vi "Get Color Ramp.vi"(9 "Number of Colors":i32, 11 "Color Ramp Array":u32[](array[colorbox])) -> (3 "RGB Array":u32[](array[colorbox]))   [LabVIEW 2020, in "3D Plot.lvclass"]
uses:
  <vilib>/Math Plots/3D Math Plots/3D Plot/3D Plot/3D Plot.lvclass
  <vilib>/Utility/colorconv.llb/Color to RGB.vi
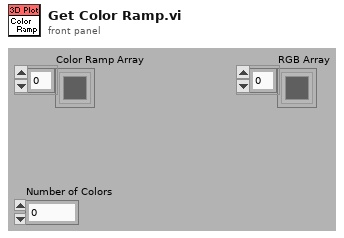
[diagram p1: front panel]
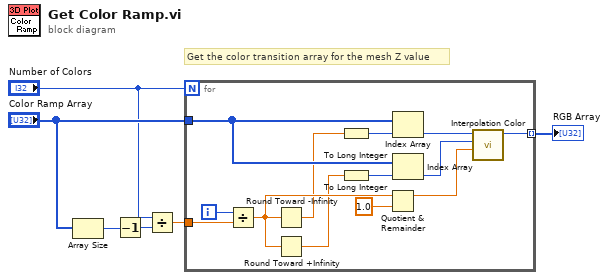
[diagram p0: block diagram]
diagram:
  # "Get the color transition array for the mesh Z value"
  n1 = Array Size(array="Color Ramp Array") -> (size(s)=w5:i32)
  n2 = Decrement(x=w5) -> (x-1=w3:i32)
  n3 = Divide(x="Number of Colors", y=w3) -> (x/y=w4:dbl)
  n4 = for {
    N: "Number of Colors" -> [_]
    tunnel: "Color Ramp Array" -> [w18]
    tunnel: w4 -> [w19]
    tunnel: [w11] -> w1 mode=indexing
    i -> [w16]
    n5 = Divide(x=w16, y=w19) -> (x/y=w15:dbl)
    n6 = Round Toward -Infinity(1:w15) -> (0:w7:dbl)
    n7 = Round Toward +Infinity(x=w15) -> (ceil(x): smallest int >= x=w8:dbl)
    n8 = To Long Integer(number=w7) -> (32bit integer=w10:i32)
    n9 = To Long Integer(number=w8) -> (32bit integer=w9:i32)
    n10 = Quotient & Remainder(x=w15, y=1.0) -> (x-y*floor(x/y)=w12:dbl)  [unwired: 1 out]
    n11 = Index Array(array=w18, index=w10) -> (element=w14:u32)
    n12 = Index Array(array=w18, index=w9) -> (element=w13:u32)
    n13 = call <vilib>:"Interpolation Color.vi"("Interpolation Value"=w12, "Input Color2"=w13, "Input Color1"=w14) -> ("Output Color"=w11:u32)  [unwired: 8 out]
  }
  "RGB Array" <- w1
